vi "Format Crosstalk Table in uA.vi"(0 "Header":string[](array[string])=["CH1", "CH2", "CH3", "CH4", "CH5", "CH6", "CH7", "CH8", "CH9", "CH10", "CH11", "CH12", "CH13", "CH14", "CH15", "CH16", "CH17", "CH18", "CH19", "CH20", "CH21", "CH22", "CH23", "CH24", "CH25"], 5 "Data Table":dbl[][](array[numeric])=[[1.0, 2.0, 3.0, 4.0, 5.0, 6.0, 7.0, 8.0, 9.0, 10.0, 11.0, 12.0, 13.0, 14.0, 15.0, 16.0, 17.0, 18.0, 19.0, 20.0, 21.0, 22.0, 23.0, 24.0, 25.0], [2.0, 999.0, 0.0, 0.0, 0.0, 0.0, 0.0, 0.0, 0.0, 0.0, 0.0, 0.0, 0.0, 0.0, 0.0, 0.0, 0.0, 0.0, 0.0, 0.0, 0.0, 0.0, 0.0, 0.0, 0.0], [3.0, 0.0, 999.0, 0.0, 0.0, 0.0, 0.0, 0.0, 0.0, 0.0, 0.0, 0.0, 0.0, 0.0, 0.0, 0.0, 0.0, 0.0, 0.0, 0.0, 0.0, 0.0, 0.0, 0.0, 0.0], [4.0, 0.0, 0.0, 999.0, 0.0, 0.0, 0.0, 0.0, 0.0, 0.0, 0.0, 0.0, 0.0, 0.0, 0.0, 0.0, 0.0, 0.0, 0.0, 0.0, 0.0, 0.0, 0.0, 0.0, 0.0], [5.0, 0.0, 0.0, 0.0, 999.0, 0.0, 0.0, 0.0, 0.0, 0.0, 0.0, 0.0, 0.0, 0.0, 0.0, 0.0, 0.0, 0.0, 0.0, 0.0, 0.0, 0.0, 0.0, 0.0, 0.0], [6.0, 0.0, 0.0, 0.0, 0.0, 999.0, 0.0, 0.0, 0.0, 0.0, 0.0, 0.0, 0.0, 0.0, 0.0, 0.0, 0.0, 0.0, 0.0, 0.0, 0.0, 0.0, 0.0, 0.0, 0.0], [7.0, 0.0, 0.0, 0.0, 0.0, 0.0, 999.0, 0.0, 0.0, 0.0, 0.0, 0.0, 0.0, 0.0, 0.0, 0.0, 0.0, 0.0, 0.0, 0.0, 0.0, 0.0, 0.0, 0.0, 0.0], [8.0, 0.0, 0.0, 0.0, 0.0, 0.0, 0.0, 999.0, 0.0, 0.0, 0.0, 0.0, 0.0, 0.0, 0.0, 0.0, 0.0, 0.0, 0.0, 0.0, 0.0, 0.0, 0.0, 0.0, 0.0], [9.0, 0.0, 0.0, 0.0, 0.0, 0.0, 0.0, 0.0, 999.0, 0.0, 0.0, 0.0, 0.0, 0.0, 0.0, 0.0, 0.0, 0.0, 0.0, 0.0, 0.0, 0.0, 0.0, 0.0, 0.0], [10.0, 0.0, 0.0, 0.0, 0.0, 0.0, 0.0, 0.0, 0.0, 999.0, 0.0, 0.0, 0.0, 0.0, 0.0, 0.0, 0.0, 0.0, 0.0, 0.0, 0.0, 0.0, 0.0, 0.0, 0.0], [11.0, 0.0, 0.0, 0.0, 0.0, 0.0, 0.0, 0.0, 0.0, 0.0, 999.0, 0.0, 0.0, 0.0, 0.0, 0.0, 0.0, 0.0, 0.0, 0.0, 0.0, 0.0, 0.0, 0.0, 0.0], [12.0, 0.0, 0.0, 0.0, 0.0, 0.0, 0.0, 0.0, 0.0, 0.0, 0.0, 999.0, 0.0, 0.0, 0.0, 0.0, 0.0, 0.0, 0.0, 0.0, 0.0, 0.0, 0.0, 0.0, 0.0], [13.0, 0.0, 0.0, 0.0, 0.0, 0.0, 0.0, 0.0, 0.0, 0.0, 0.0, 0.0, 999.0, 0.0, 0.0, 0.0, 0.0, 0.0, 0.0, 0.0, 0.0, 0.0, 0.0, 0.0, 0.0], [14.0, 0.0, 0.0, 0.0, 0.0, 0.0, 0.0, 0.0, 0.0, 0.0, 0.0, 0.0, 0.0, 999.0, 0.0, 0.0, 0.0, 0.0, 0.0, 0.0, 0.0, 0.0, 0.0, 0.0, 0.0], [15.0, 0.0, 0.0, 0.0, 0.0, 0.0, 0.0, 0.0, 0.0, 0.0, 0.0, 0.0, 0.0, 0.0, 999.0, 0.0, 0.0, 0.0, 0.0, 0.0, 0.0, 0.0, 0.0, 0.0, 0.0], [16.0, 0.0, 0.0, 0.0, 0.0, 0.0, 0.0, 0.0, 0.0, 0.0, 0.0, 0.0, 0.0, 0.0, 0.0, 999.0, 0.0, 0.0, 0.0, 0.0, 0.0, 0.0, 0.0, 0.0, 0.0], [17.0, 0.0, 0.0, 0.0, 0.0, 0.0, 0.0, 0.0, 0.0, 0.0, 0.0, 0.0, 0.0, 0.0, 0.0, 0.0, 999.0, 0.0, 0.0, 0.0, 0.0, 0.0, 0.0, 0.0, 0.0], [18.0, 0.0, 0.0, 0.0, 0.0, 0.0, 0.0, 0.0, 0.0, 0.0, 0.0, 0.0, 0.0, 0.0, 0.0, 0.0, 0.0, 999.0, 0.0, 0.0, 0.0, 0.0, 0.0, 0.0, 0.0], [19.0, 0.0, 0.0, 0.0, 0.0, 0.0, 0.0, 0.0, 0.0, 0.0, 0.0, 0.0, 0.0, 0.0, 0.0, 0.0, 0.0, 0.0, 999.0, 0.0, 0.0, 0.0, 0.0, 0.0, 0.0], [20.0, 0.0, 0.0, 0.0, 0.0, 0.0, 0.0, 0.0, 0.0, 0.0, 0.0, 0.0, 0.0, 0.0, 0.0, 0.0, 0.0, 0.0, 0.0, 999.0, 0.0, 0.0, 0.0, 0.0, 0.0], [21.0, 0.0, 0.0, 0.0, 0.0, 0.0, 0.0, 0.0, 0.0, 0.0, 0.0, 0.0, 0.0, 0.0, 0.0, 0.0, 0.0, 0.0, 0.0, 0.0, 999.0, 0.0, 0.0, 0.0, 0.0], [22.0, 0.0, 0.0, 0.0, 0.0, 0.0, 0.0, 0.0, 0.0, 0.0, 0.0, 0.0, 0.0, 0.0, 0.0, 0.0, 0.0, 0.0, 0.0, 0.0, 0.0, 999.0, 0.0, 0.0, 0.0], [23.0, 0.0, 0.0, 0.0, 0.0, 0.0, 0.0, 0.0, 0.0, 0.0, 0.0, 0.0, 0.0, 0.0, 0.0, 0.0, 0.0, 0.0, 0.0, 0.0, 0.0, 0.0, 999.0, 0.0, 0.0], [24.0, 0.0, 0.0, 0.0, 0.0, 0.0, 0.0, 0.0, 0.0, 0.0, 0.0, 0.0, 0.0, 0.0, 0.0, 0.0, 0.0, 0.0, 0.0, 0.0, 0.0, 0.0, 0.0, 999.0, 0.0], [25.0, 0.0, 0.0, 0.0, 0.0, 0.0, 0.0, 0.0, 0.0, 0.0, 0.0, 0.0, 0.0, 0.0, 0.0, 0.0, 0.0, 0.0, 0.0, 0.0, 0.0, 0.0, 0.0, 0.0, 999.0]]) -> (4 "HTML-formatted Table":string, 8 "Table Passed?":bool, 10 "Pass Count":dbl=nan, 15 "Amplitudes 2-D w/Headers":string[][](array[string]))   [LabVIEW 2010]
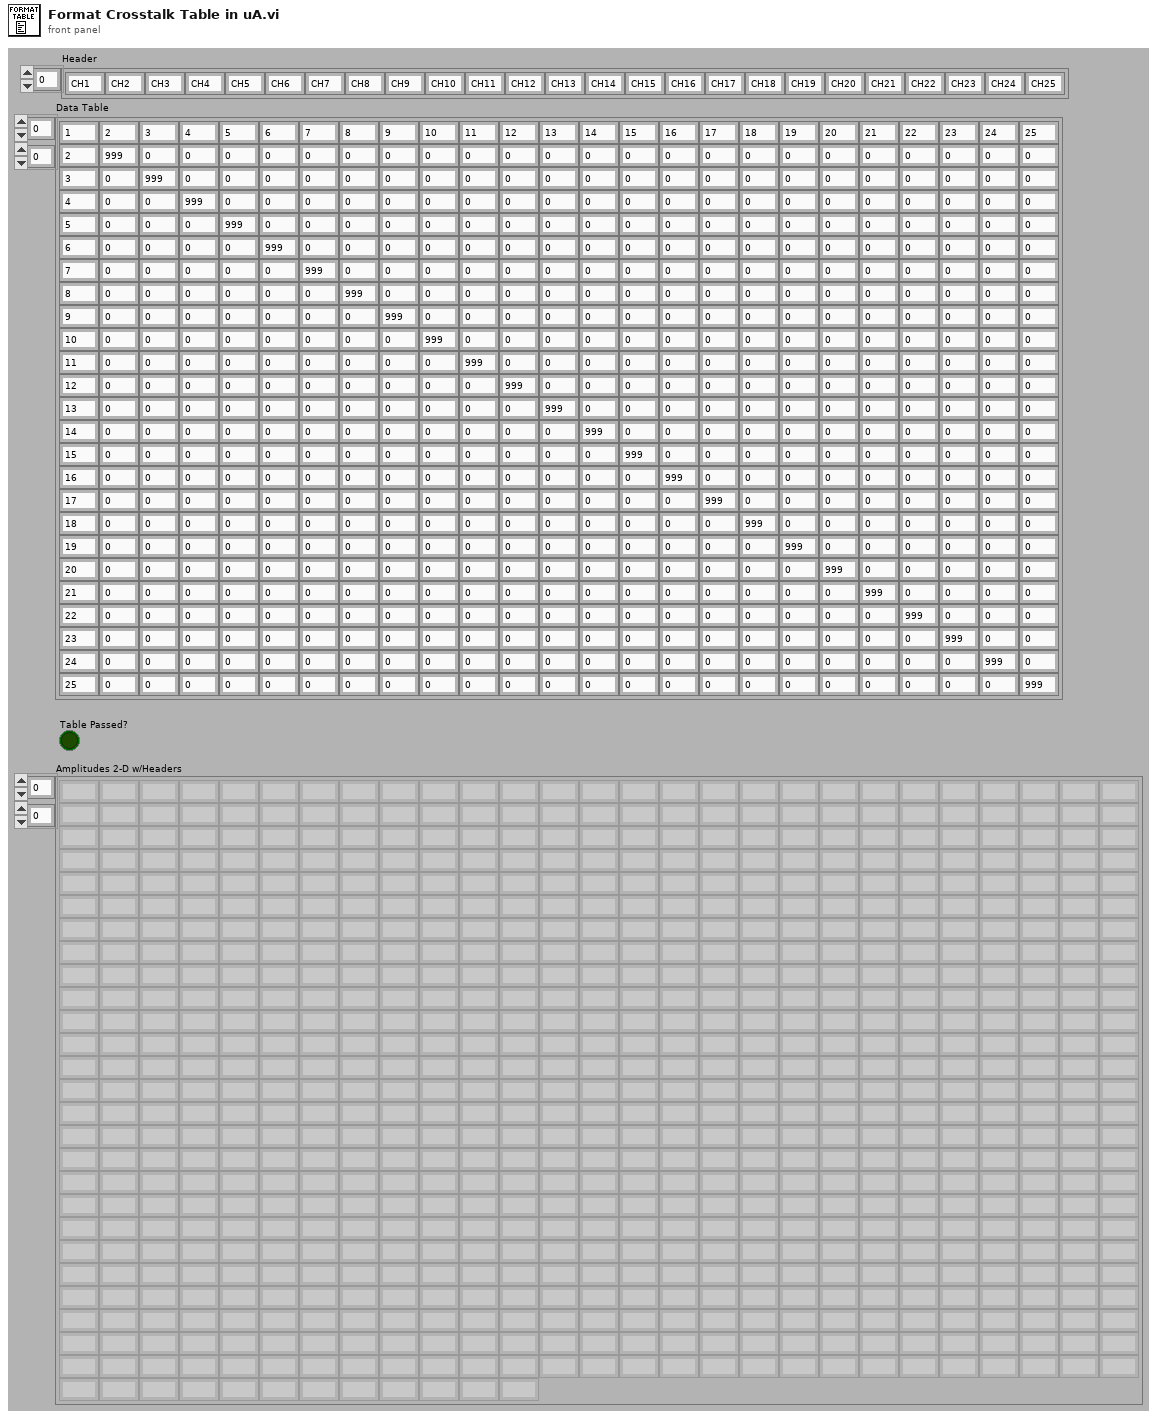
[diagram p1: front panel]
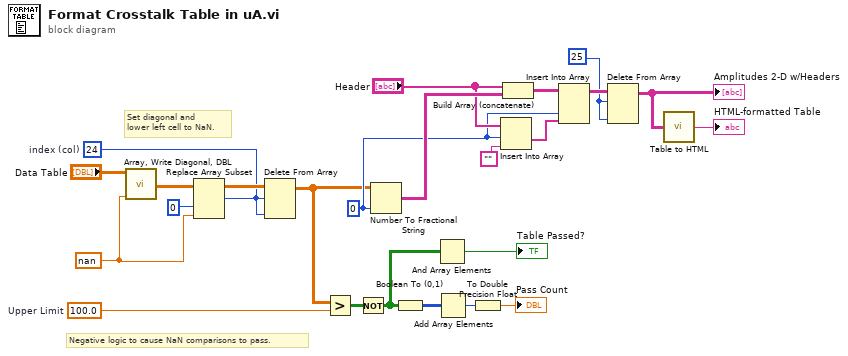
[diagram p0: block diagram]
diagram:
  w1 = 25 ("length")
  w12 = nan ("element")
  w2 = 24  # index (col)
  w17 = 100.0  # Upper Limit
  w8 = 0 ("precision (6)")
  # "Negative logic to cause NaN comparisons to pass."
  # "Set diagonal and\nlower left cell to NaN."
  n1 = call "Array, Write Diagonal, DBL.vi"("diagonal (1)"=w12, "array in"="Data Table") -> ("array out"=w3:dbl[][])  [unwired: 2 in]
  n2 = Replace Array Subset(array=w3, new element=w12, index (row)=w2, index (col)=0 ("disabled index (col)")) -> (w5:dbl[][])
  n3 = Delete From Array(array=w5, length=w2, index (col)=w2) -> (array with subset deleted=w4:dbl[][])  [unwired: 1 in, 1 out]
  n4 = Greater?(x=w4, y=w17) -> (0:w11:bool[][])
  n5 = Not(x=w11) -> (.not. x?=w9:bool[][])
  n6 = Number To Fractional String(number=w4, precision (6)=w8) -> (F-format string=w24:string[][])  [unwired: 2 in]
  n7 = Boolean To (0,1)(Boolean=w9) -> (0, 1=w10:i16[][])
  n8 = And Array Elements(Boolean array=w9) -> (logical AND=→"Table Passed?":bool)
  n9 = Add Array Elements(numeric array=w10) -> (sum=w16:i16)
  n10 = To Double Precision Float(number=w16) -> (double precision float=→"Pass Count":dbl)
  n11 = Insert Into Array(array="Header", index=w8, new element="") -> (w18:string[])
  n12 = Build Array (concatenate)("Header", w24) -> (w21:string[][])
  n13 = Insert Into Array(array=w21, index (col)=w8, new element=w18) -> (w7:string[][])  [unwired: 1 in]
  n14 = Delete From Array(array=w7, length=w1, index (col)=w1) -> (array with subset deleted=w6:string[][])  [unwired: 1 in, 1 out]
  "Amplitudes 2-D w/Headers" <- w6
  n15 = call "Table to HTML.vi"("Table"=w6) -> ("HTML-formatted Table"=→"HTML-formatted Table":string)
